vi "Laurel Commands.vi"(8 "Error In":errorcluster, 11 "Laurel Serial Commands":T1) -> (0 "Error Out":errorcluster, 2 "Send Command out":string)   [LabVIEW 2020]
uses:
  Type Definitions/Laurel Serial Commands.ctl
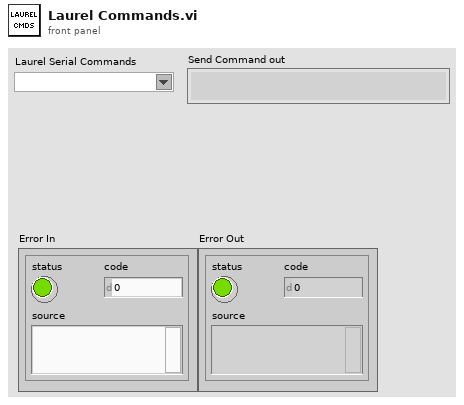
[diagram p1: front panel]
types:
  T1 = typedef "Laurel Serial Commands.ctl" = string
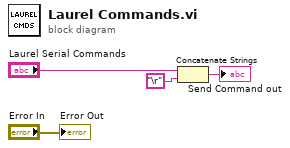
[diagram p0: block diagram]
diagram:
  n1 = Concatenate Strings("Laurel Serial Commands", "\r") -> (→"Send Command out":string)
  "Error Out" <- "Error In"
